vi "Day 16-1.vi"() -> ()   [LabVIEW 2020]
uses:
  Packet/Packet.lvclass
panel:
  out "Value":i64
  out "Version Sum":i32
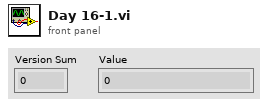
[diagram p1: front panel]
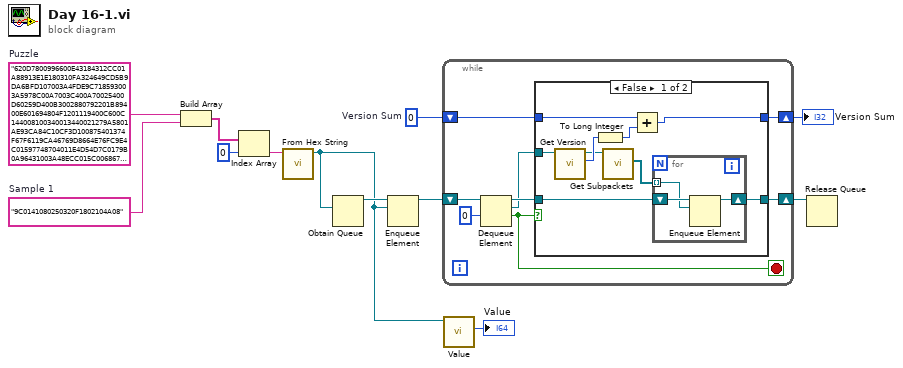
[diagram p0: block diagram]
diagram:
  w4 = 0  # Version Sum
  w11 = "9C0141080250320F1802104A08"  # Sample 1
  w12 = "620D7800996600E43184312CC01A88913E1E180310FA324649CD5B9DA6BFD107003A4FDE9C718593003A5978C00A7003C400A70025400D60259D400B3002880792201B89400E601694804F1201119400C600C144008100340013440021279A5801AE93CA84C10CF3D100875401374F67F6119CA46769D8664E76FC9E4C01597748704011E4D54D7C0179B0A96431003A48ECC015C0068670FA7EF1BC5166CE440239EFC226F228129E8C1D6633596716E7D4840129C4C8CA8017FCFB943699B794210CAC23A612012EB40151006E2D4678A4200EC548CF12E4FDE9BD4A5227C600F80021D08219C1A00043A27C558AA200F4788C91A1002C893AB24F722C129BDF5121FA8011335868F1802AE82537709999796A7176254A72F8E9B9005BD600A4FD372109FA6E42D1725EDD..."  # Puzzle
  n1 = Build Array(w12, w11) -> (w10:string[])
  n2 = Index Array(array=w10, index=0) -> (element=w8:string)
  n3 = call "From Hex String.vi"("String"=w8) -> ("Packet out"=w2:refnum<class "Packet.lvclass">)  [unwired: 9 in, 1 out]
  n4 = Obtain Queue(element data type=w2) -> (queue out=w7:refnum<queue>)  [unwired: 4 in, 2 out]
  n5 = Enqueue Element(queue=w7, element=w2) -> (queue out=w6:refnum<queue>)  [unwired: 2 in, 2 out]
  n6 = while {
    shift-right: [w15] -> w5
    shift-left: w6 -> [w20]
    shift-right: [w13] -> w3
    shift-left: w4 -> [w14]
    stop <- w17 stop-if-true
    n7 = Dequeue Element(queue=w20, timeout in ms (-1)=0) -> (queue out=w18:refnum<queue>, element=w16:refnum<class "Packet.lvclass">, timed out?=w17:bool)  [unwired: 1 in, 1 out]
    n8 = case shown="False" w17 {
      tunnel: w18 -> [w23 w34]
      tunnel: w16 -> [w29 _]
      tunnel: [w21 w34] -> w15
      tunnel: w14 -> [w27 w33]
      tunnel: [w25 w33] -> w13
      frame False {
        n9 = call "Get Version.vi"("Packet in"=w29) -> ("Version"=w28:u8, "Packet out"=w24:refnum<class "Packet.lvclass">)  [unwired: 8 in, 1 out]
        n10 = To Long Integer(number=w28) -> (32bit integer=w26:i32)
        n11 = call-dynamic "Get Subpackets.vi"("Packet in"=w24) -> ("Subpackets"=w22:refnum<class "Packet.lvclass">[])  [unwired: 8 in, 2 out]
        n12 = Add(x=w27, y=w26) -> (x+y=w25:i32)
        n13 = for {
          shift-right: [w31] -> w21
          shift-left: w23 -> [w32]
          tunnel: w22 -> [w30] mode=indexing
          n14 = Enqueue Element(queue=w32, element=w30) -> (queue out=w31:refnum<queue>)  [unwired: 2 in, 2 out]
        }
      }
      frame True {
      }
    }
  }
  "Version Sum" <- w3
  n15 = call-dynamic "Value.vi"("Packet in"=w2) -> ("Value"=→"Value":i64)  [unwired: 8 in, 2 out]
  n16 = Release Queue(queue=w5) -> ()  [unwired: 2 in, 3 out]
